vi "GetConpaneImage.vi"(4 "Error in":errorcluster caption="Error in (no error)", 5 "Color Outputs (T)":bool=TRUE, 6 "Color Inputs (T)":bool=TRUE, 7 "VI Ref":refnum<vi>) -> (0 "Error out":errorcluster, 2 "VI connector pane image":picture, 3 "dup VI Ref":refnum<vi>)   [LabVIEW 2025, in "XNode Support.lvlib"]
doc: "Gets the <B>VI connector pane image</B> from the VI specified by <B>VI reference</B>.\n\nModified from a VI by\nSteen Schmidt, GPower, 21/2 2013"
uses:
  XNode Support.lvlib
  <vilib>/Utility/miscctls.llb/LVRectTypeDef.ctl
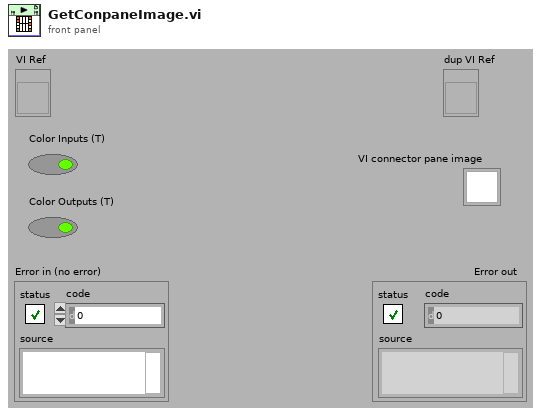
[diagram p1: front panel]
types:
  T1 = typedef "LVRectTypeDef.ctl" = cluster{"Left":i16, "Top":i16, "Right":i16, "Bottom":i16}
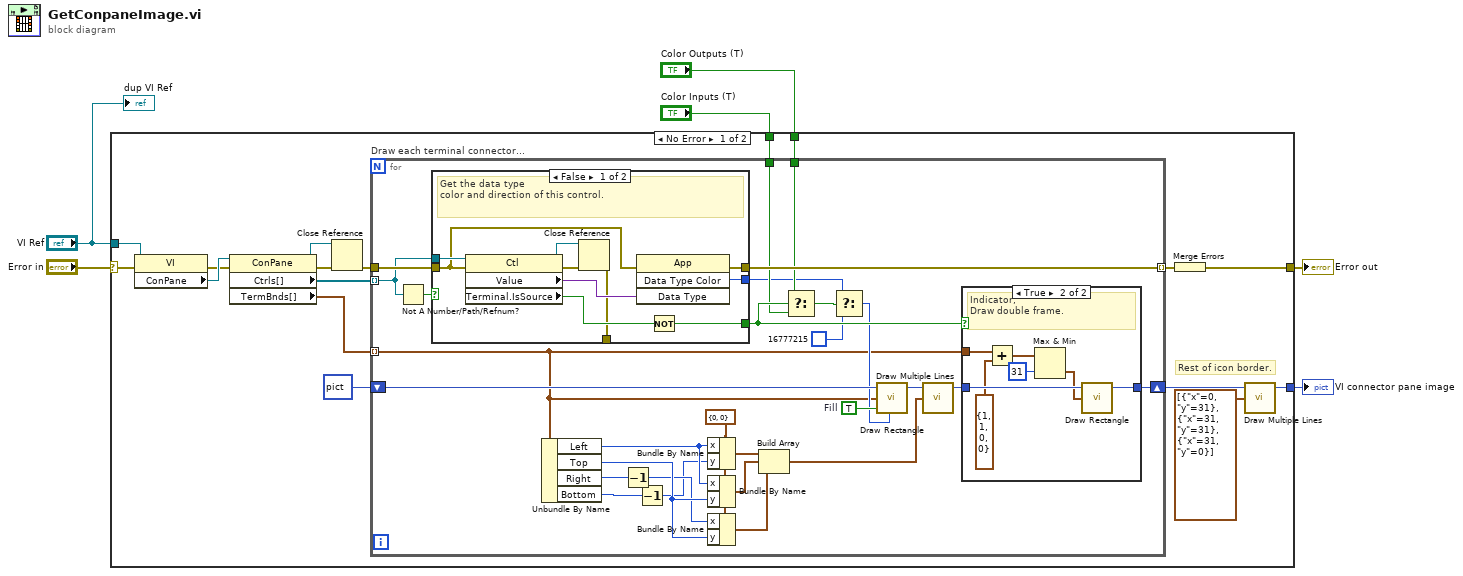
[diagram p0: block diagram]
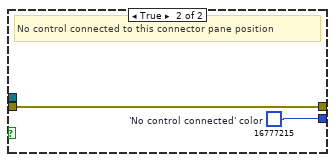
[diagram p2: hidden frame]
diagram:
  n1 = case shown="No Error" "Error in" {
    selector: "Error in" -> [w16 w72]
    tunnel: [w7 w72] -> w6
    tunnel: "VI Ref" -> [w23 _]
    tunnel: [w12 _] -> w4
    tunnel: "Color Outputs (T)" -> [w9 _]
    tunnel: "Color Inputs (T)" -> [w8 _]
    frame No Error {
      # "Rest of icon border."
      n2 = property class="VI"(reference=w23, error in=w16) -> (error out=w21:errorcluster, "ConPane"=w22:refnum<vi>)  [unwired: 1 out]
      n3 = property class="ConPane"(reference=w22, error in=w21) -> (reference out=w19:refnum<vi>, error out=w20:errorcluster, "Ctrls[]"=w18:refnum<vi>[], "TermBnds[]"=w14:T1[])
      n4 = Close Reference(reference=w19, error in (no error)=w20) -> (error out=w17:errorcluster)
      n5 = for "Draw each terminal connector..." {
        tunnel: w14 -> [w24] mode=indexing
        tunnel: w18 -> [w49] mode=indexing
        shift-right: [w42] -> w13
        shift-left: picture data[5B] ("empty picture") -> [w38]
        tunnel: w9 -> [w30]
        tunnel: w8 -> [w29]
        tunnel: w17 -> [w51]
        tunnel: [w48] -> w15 mode=indexing
        w32 = TRUE  # Fill
        w37 = cluster{"x":i16, "y":i16} {"x"=0, "y"=0}
        n6 = Not A Number/Path/Refnum?(number/path/refnum=w49) -> (NaN/Path/Refnum?=w50:bool)
        n7 = case shown="False" w50 {
          tunnel: w51 -> [w52 w62]
          tunnel: w49 -> [w61 _]
          tunnel: [w58 w62] -> w48
          tunnel: [w57 w63] -> w27
          tunnel: [w55 _] -> w31
          tunnel: [w53 _] -> _
          frame False {
            # "Get the data type\ncolor and direction of this control."
            n8 = property class="Ctl"(reference=w61, error in=w52) -> (reference out=w59:refnum<vi>, error out=w60:errorcluster, "Value"=w54:variant, "Terminal.IsSource"=w56:bool)
            n9 = Close Reference(reference=w59, error in (no error)=w60) -> (error out=w53:errorcluster)
            n10 = invoke class="App" method="Data Type Color"(error in=w52, "Data Type"=w54) -> (error out=w58:errorcluster, "Data Type Color"=w57:u32)  [unwired: 2 in, 2 out]
            n11 = Not(x=w56) -> (.not. x?=w55:bool)
          }
          frame True {
            w63 = u32 16777215  # 'No control connected' color
            # "No control connected to this connector pane position"
          }
        }
        n12 = Unbundle By Name(w24) -> ("Left"=w46:i16, "Top"=w44:i16, "Right"=w45:i16, "Bottom"=w47:i16)
        n13 = Decrement(x=w45) -> (x-1=w41:i16)
        n14 = Decrement(x=w47) -> (x-1=w40:i16)
        n15 = Bundle By Name(cluster=w37, "x"=w46, "y"=w40) -> (w36:cluster{"x":i16, "y":i16})
        n16 = Bundle By Name(cluster=w37, "x"=w46, "y"=w44) -> (w35:cluster{"x":i16, "y":i16})
        n17 = Bundle By Name(cluster=w37, "x"=w41, "y"=w44) -> (w34:cluster{"x":i16, "y":i16})
        n18 = Build Array(w36, w35, w34) -> (w33:cluster{"x":i16, "y":i16}[])
        n19 = Select(t=w30, s=w31, f=w29) -> (s? t:f=w28:bool)
        n20 = Select(t=w27, s=w28, f=u32 16777215) -> (s? t:f=w26:u32)
        n21 = call <vilib>:"Draw Rectangle.vi"("picture"=w38, "rect"=w24, "fill?(F)"=w32, "color(black)"=w26) -> ("new picture"=w39:picture)  [unwired: 5 in]
        n22 = call <vilib>:"Draw Multiple Lines.vi"("picture"=w39, "line endpoints"=w33) -> ("new picture"=w43:picture)  [unwired: 7 in]
        n23 = case "Is indicator?" shown="True" w31 {
          tunnel: w43 -> [w64 w71]
          tunnel: [w64 w70] -> w42
          tunnel: w24 -> [_ w69]
          frame False {
          }
          frame True {
            # "Indicator;\nDraw double frame."
            n24 = Add(x=w69, y=T1 {"Left"=1, "Top"=1, "Right"=0, "Bottom"=0} ("Rectangle")) -> (x+y=w67:T1)
            n25 = Max & Min(x=w67, y=i16 31 ("Left")) -> (min(x,y)=w66:T1)  [unwired: 1 out]
            n26 = call <vilib>:"Draw Rectangle.vi"("picture"=w71, "rect"=w66) -> ("new picture"=w70:picture)  [unwired: 7 in]
          }
        }
      }
      n27 = Merge Errors(w15) -> (w7:errorcluster)
      n28 = call <vilib>:"Draw Multiple Lines.vi"("picture"=w13, "line endpoints"=cluster{"x":i16, "y":i16}[] [{"x"=0, "y"=31}, {"x"=31, "y"=31}, {"x"=31, "y"=0}]) -> ("new picture"=w12:picture)  [unwired: 7 in]
    }
    frame Error {
    }
  }
  "VI connector pane image" <- w4
  "Error out" <- w6
  "dup VI Ref" <- "VI Ref"
